vi "Init OI.vi"(8 "error in":errorcluster, 10 "control ref cluster":T1, 11 "VI ref":refnum<vi>) -> (0 "error out":errorcluster)   [LabVIEW 2018]
uses:
  Ctls/Types of Controls.ctl
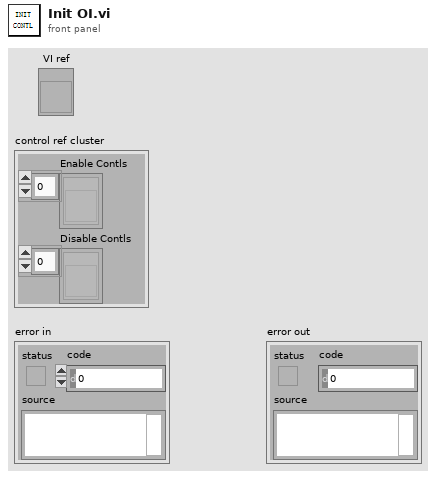
[diagram p1: front panel]
types:
  T1 = typedef "Types of Controls.ctl" = cluster{"Enable Contls":refnum<vi>[], "Disable Contls":refnum<vi>[]}
  T2 = enum8{"Enabled", "Disabled", "Disabled and Grayed Out"}
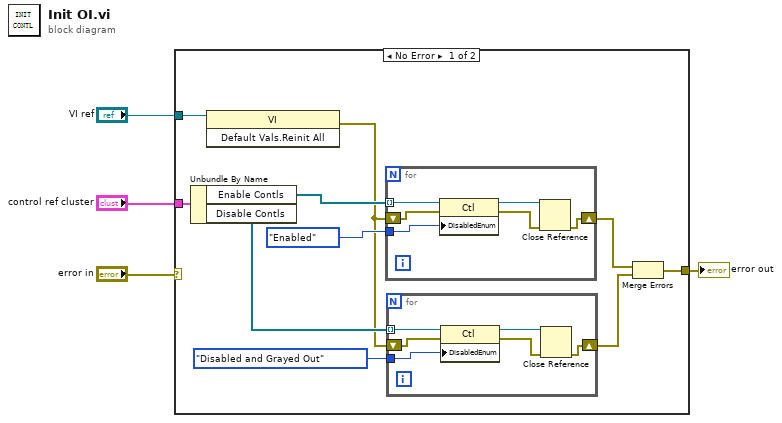
[diagram p0: block diagram]
diagram:
  n1 = case shown="No Error" "error in" {
    selector: "error in" -> [_ w27]
    tunnel: "VI ref" -> [w14 _]
    tunnel: "control ref cluster" -> [w13 _]
    tunnel: [w5 w27] -> w1
    frame No Error {
      n2 = Unbundle By Name(w13) -> ("Enable Contls"=w12:refnum<vi>[], "Disable Contls"=w10:refnum<vi>[])
      n3 = invoke class="VI" method="Default Vals.Reinit All"(reference=w14) -> (error out=w8:errorcluster)  [unwired: 2 in, 2 out]
      n4 = for {
        tunnel: w12 -> [w26] mode=indexing
        shift-right: [w21] -> w7
        shift-left: w8 -> [w25]
        tunnel: T2."Enabled" ("Disabled") -> [w24]
        n5 = property class="Ctl"(reference=w26, error in=w25, "DisabledEnum"=w24) -> (reference out=w23:refnum<vi>, error out=w22:errorcluster)
        n6 = Close Reference(reference=w23, error in (no error)=w22) -> (error out=w21:errorcluster)
      }
      n7 = for {
        tunnel: w10 -> [w20] mode=indexing
        shift-right: [w15] -> w6
        shift-left: w8 -> [w19]
        tunnel: T2."Disabled and Grayed Out" ("Disabled") -> [w18]
        n8 = property class="Ctl"(reference=w20, error in=w19, "DisabledEnum"=w18) -> (reference out=w17:refnum<vi>, error out=w16:errorcluster)
        n9 = Close Reference(reference=w17, error in (no error)=w16) -> (error out=w15:errorcluster)
      }
      n10 = Merge Errors(w7, w6) -> (w5:errorcluster)
    }
    frame Error {
    }
  }
  "error out" <- w1
